vi "ControlMotorTest_Connect.vi"() -> ()   [LabVIEW 2018]
panel:
  out "通信成功？":bool
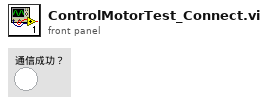
[diagram p1: front panel]
types:
  T1 = typedef "控制电机指令枚举器.ctl" = enum16{"归0", "停止", "运动", "轴设置", "通信连接"}
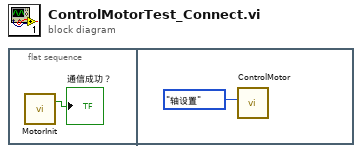
[diagram p0: block diagram]
diagram:
  n1 = flat-sequence {
    frame #0 {
      n2 = call "MotorInit.vi"() -> ("通信成功？"=→"通信成功？":bool)  [unwired: 2 in, 1 out]
    }
    frame #1 {
      n3 = call "ControlMotor.vi"("控制电机指令"=控制电机指令枚举器."轴设置") -> ()  [unwired: 7 in, 1 out]
    }
  }
